vi "Exercise 1 Solution.vi"() -> ()   [LabVIEW 2019]
panel:
  out "String":string="Hello, World!"
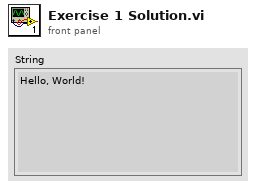
[diagram p1: front panel]
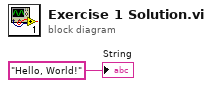
[diagram p0: block diagram]
diagram:
  "String" <- "Hello, World!"
